vi "Update Unicode Controls Async.vi"(9 "Stop Event":refnum<user-event>, 10 "Value Change Event":refnum<user-event>, 11 "String Refs":refnum<vi>[](array[refnum])) -> ()   [LabVIEW 2020, in "G-Unicode.lvlib"]
doc: "Update the controls in <b>String Refs</b> with the correct unicode value when a user types text.\n\nAll controls in <b>String Refs</b> will have their Update While Typing? and Force Unicode Text properties set True."
uses:
  G-Unicode.lvlib
  6a2c997b-0cb1-4cc4-a80f-efd7fbe50132.vi
  User Interface/Write String.vi
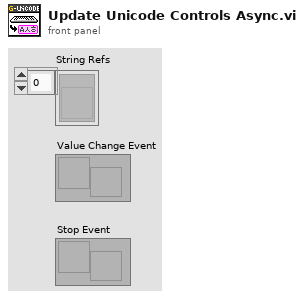
[diagram p1: front panel]
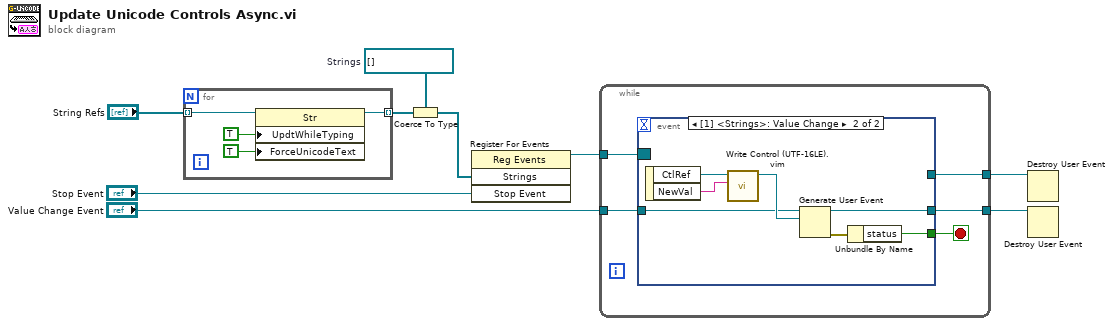
[diagram p0: block diagram]
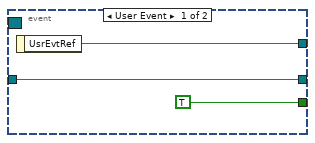
[diagram p2: hidden frame]
diagram:
  w5 = refnum<vi>[] []  # Strings
  n1 = for {
    tunnel: "String Refs" -> [w10] mode=indexing
    tunnel: [w12] -> w8 mode=indexing
    n2 = property class="Str"(reference=w10, "UpdtWhileTyping"=TRUE ("Update While Typing?"), "ForceUnicodeText"=TRUE ("Force Unicode Text")) -> (reference out=w12:refnum<vi>)  [unwired: 1 in, 1 out]
  }
  n3 = Coerce To Type(0:w8, 1:w5) -> (2:w6:refnum<vi>[])
  n4 = register-events(w6, "Stop Event") -> (reference out=w9:refnum<event-registration>)  [unwired: 2 in, 1 out]
  n5 = while {
    tunnel: w9 -> [w18]
    tunnel: [w16] -> w2
    tunnel: "Value Change Event" -> [w15]
    tunnel: [w14] -> w1
    stop <- w17 stop-if-true
    n6 = event shown="[1] <Strings>: Value Change" {
      selector: w18 -> [_ _]
      dyn-events: _ -> [_ _]
      timeout: _ -> [_ _]
      tunnel: [TRUE w25] -> w17
      tunnel: [w20 w22] -> w16
      tunnel: w15 -> [w20 w23]
      tunnel: [w19 _] -> w14
      event User Event {
        n7 = event-data() -> ("UsrEvtRef"=w19:refnum<user-event>)  [unwired: 1 in]
      }
      event Value Change {
        n8 = event-data() -> ("CtlRef"=w28:refnum<vi>, "NewVal"=w27:string)  [unwired: 1 in]
        n9 = call "Write Control (UTF-16LE).vim"("UTF-16LE String"=w27, "Control Ref"=w28) -> ("Control Ref dup"=w24:refnum<vi>)  [unwired: 8 in, 1 out]
        n10 = Generate User Event(user event=w23, event data cluster=w24) -> (user event out=w22:refnum<user-event>, error out=w26:errorcluster)  [unwired: 2 in]
        n11 = Unbundle By Name(w26) -> ("status"=w25:bool)
      }
    }
  }
  n12 = Destroy User Event(user event=w1) -> ()  [unwired: 1 in, 1 out]
  n13 = Destroy User Event(user event=w2) -> ()  [unwired: 1 in, 1 out]
